vi "pin_mapping.vi"() -> ()   [LabVIEW 2022 SP3]
uses:
  <vilib>/Utility/file.llb/Read Delimited Spreadsheet (string).vi
  <vilib>/Utility/file.llb/Write Delimited Spreadsheet (string).vi
panel:
  out "all rows 2":string[][](array[string])
  out "all rows":string[][](array[string])
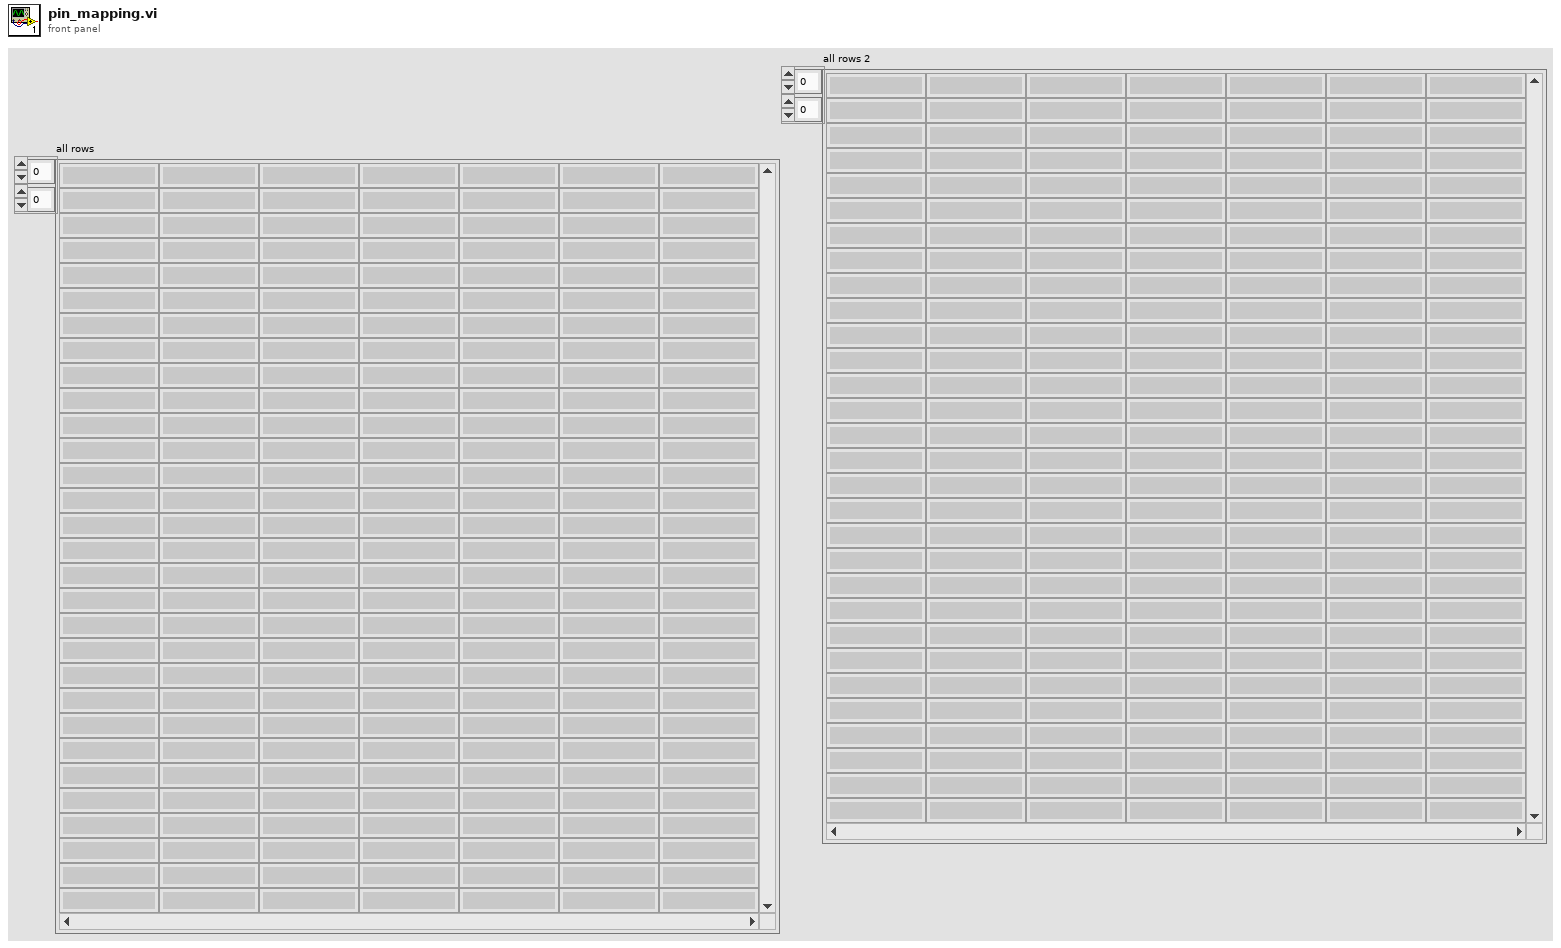
[diagram p1: front panel]
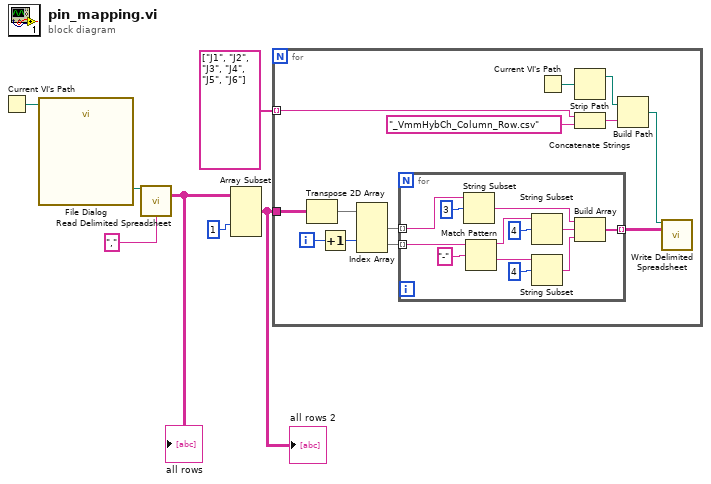
[diagram p0: block diagram]
diagram:
  n1 = Current VI's Path() -> (path=w6:path)
  n2 = call "File Dialog"("start path"=w6) -> ("selected path"=w2:path)  [unwired: 11 in, 3 out]
  n3 = call-poly <vilib>:"Read Delimited Spreadsheet.vi"("file path (dialog if empty)"=w2, "delimiter (\\t)"="," ("delimiter (\\t)")) -> ("all rows"=w3:string[][])  [unwired: 8 in, 5 out]
  "all rows" <- w3
  n4 = Array Subset(array=w3, index (col)=1 ("index")) -> (w1:string[][])  [unwired: 3 in]
  "all rows 2" <- w1
  n5 = for {
    tunnel: w1 -> [w18]
    tunnel: string[] ["J1", "J2", "J3", "J4", "J5", "J6"] -> [w15] mode=indexing
    i -> [w20]
    n6 = Transpose 2D Array(2D array=w18) -> (transposed array=w19:string[][])
    n7 = Increment(x=w20) -> (x+1=w8:i32)
    n8 = Index Array(array=w19, index (row) #2=w8) -> (element #1=w17:string[], element #2=w16:string[])  [unwired: 3 in]
    n9 = for {
      tunnel: w17 -> [w31] mode=indexing
      tunnel: w16 -> [w30] mode=indexing
      tunnel: [w21] -> w12 mode=indexing
      n10 = String Subset(string=w31, offset (0)=3) -> (substring=w24:string)  [unwired: 1 in]
      n11 = Match Pattern(string=w30, regular expression="-") -> (before substring=w25:string, after substring=w27:string)  [unwired: 1 in, 2 out]
      n12 = String Subset(string=w25, offset (0)=4) -> (substring=w23:string)  [unwired: 1 in]
      n13 = String Subset(string=w27, offset (0)=4) -> (substring=w22:string)  [unwired: 1 in]
      n14 = Build Array(w24, w23, w22) -> (w21:string[])
    }
    n15 = Current VI's Path() -> (path=w10:path)
    n16 = Strip Path(path=w10) -> (stripped path=w9:path)  [unwired: 1 out]
    n17 = Concatenate Strings(w15, "_VmmHybCh_Column_Row.csv" ("string")) -> (w13:string)
    n18 = Build Path(base path=w9, name or relative path=w13) -> (appended path=w11:path)
    n19 = call-poly <vilib>:"Write Delimited Spreadsheet.vi"("file path (dialog if empty)"=w11, "2D data"=w12) -> ()  [unwired: 12 in, 2 out]
  }
